vi "Init DB-ADO.vi"(8 "error in":errorcluster, 10 "Authentication":T1, 11 "DB-ADO in":refnum<class "DB-ADO.lvclass">) -> (0 "error out":errorcluster, 3 "DB-ADO out":refnum<class "DB-ADO.lvclass">)   [LabVIEW 2014, in "hse-db.lvlib" / "DB-ADO.lvclass"]
doc: "Init a new ADO DB object."
uses:
  DB-ADO.lvclass
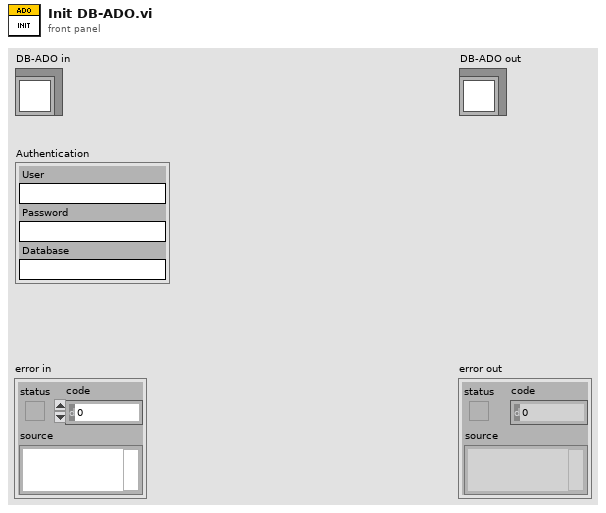
[diagram p1: front panel]
types:
  T1 = cluster{"User":string, "Password":string, "Database":string}
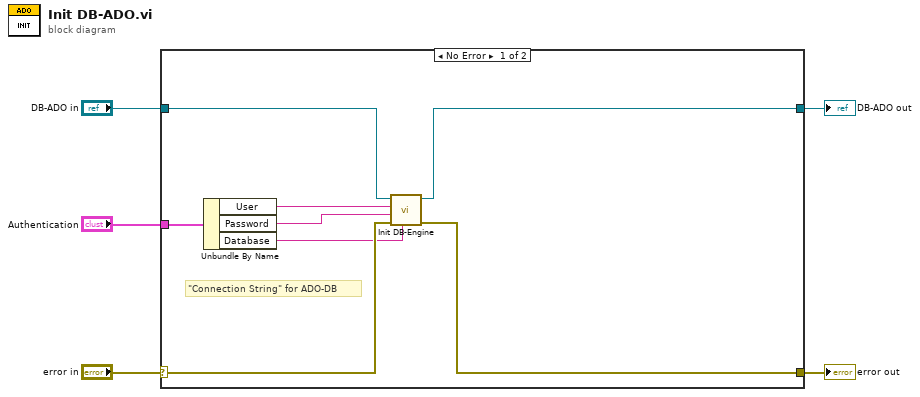
[diagram p0: block diagram]
diagram:
  n1 = case shown="No Error" "error in" {
    selector: "error in" -> [w13 w15]
    tunnel: [w12 w15] -> w4
    tunnel: [w10 w14] -> w2
    tunnel: "DB-ADO in" -> [w11 w14]
    tunnel: "Authentication" -> [w9 _]
    frame No Error {
      # "\"Connection String\" for ADO-DB"
      n2 = Unbundle By Name(w9) -> ("User"=w8:string, "Password"=w7:string, "Database"=w6:string)
      n3 = call-dynamic "Init DB-Engine.vi"("Database"=w6, "error in"=w13, "Password"=w7, "User"=w8, "DB-Engine in"=w11) -> ("error out"=w12:errorcluster, "DB-Engine out"=w10:refnum<class "DB-ADO.lvclass">)  [unwired: 5 in]
    }
    frame Error {
    }
  }
  "error out" <- w4
  "DB-ADO out" <- w2
